vi "测试定时器类.vi"() -> ()   [LabVIEW 2014]
panel:
  out "经历时间":u32
  out "定时到脉冲":bool
  out "定时到":bool
  in  "停止":bool
  in  "设定时间 s":u32
  in  "复位定时器":bool
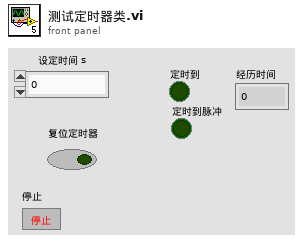
[diagram p1: front panel]
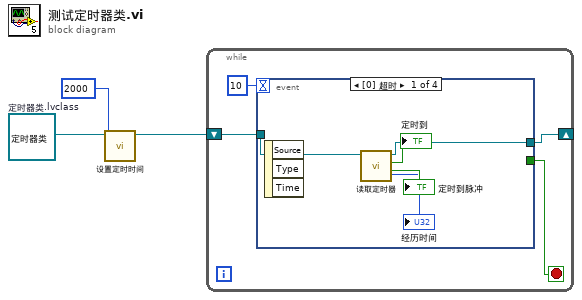
[diagram p0: block diagram]
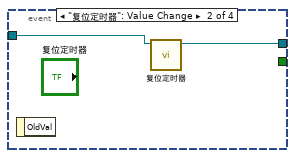
[diagram p2: hidden frame]
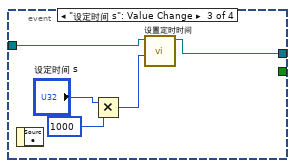
[diagram p3: hidden frame]
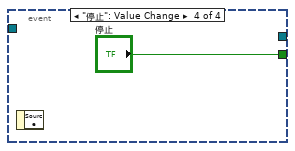
[diagram p4: hidden frame]
diagram:
  w3 = refnum<class "定时器类.lvclass"> refnum  # 定时器类.lvclass
  n1 = call-dynamic "设置定时时间.vi"("设置时间"=u32 2000, "定时器类 输入"=w3) -> ("定时器类 输出"=w1:refnum<class "定时器类.lvclass">)  [unwired: 8 in, 1 out]
  n2 = while {
    shift-right: [w5] -> _
    shift-left: w1 -> [w6]
    stop <- w4 stop-if-true
    n3 = event shown="[0] 超时" {
      selector: _ -> [_ _ _ _]
      dyn-events: _ -> [_ _ _ _]
      timeout: 10 -> [_ _ _ _]
      tunnel: w6 -> [w12 w14 w19 _]
      tunnel: [w11 w13 w15 _] -> w5
      tunnel: [_ _ _ "停止"] -> w4
      event Timeout {
        n4 = event-data() -> ()  [unwired: 1 in, 3 out]
        n5 = call-dynamic "读取定时器.vi"("定时器类 输入"=w12) -> ("定时到脉冲"=→"定时到脉冲":bool, "定时到"=→"定时到":bool, "定时器类 输出"=w11:refnum<class "定时器类.lvclass">, "经历时间"=→"经历时间":u32)  [unwired: 6 in, 1 out]
      }
      event "复位定时器": Value Change {
        n6 = event-data() -> ()  [unwired: 1 in, 1 out]
        n7 = call-dynamic "复位定时器.vi"("定时器类 输入"=w14) -> ("定时器类 输出"=w13:refnum<class "定时器类.lvclass">)  [unwired: 9 in, 1 out]
      }
      event "设定时间 s": Value Change {
        n8 = event-data() -> ()  [unwired: 1 in, 1 out]
        n9 = Multiply(x="设定时间 s", y=u32 1000) -> (x*y=w16:u32)
        n10 = call-dynamic "设置定时时间.vi"("设置时间"=w16, "定时器类 输入"=w19) -> ("定时器类 输出"=w15:refnum<class "定时器类.lvclass">)  [unwired: 8 in, 1 out]
      }
      event "停止": Value Change {
        n11 = event-data() -> ()  [unwired: 1 in, 1 out]
      }
    }
  }
